vi "VXM-MoveOneAxisToHome.vi"(8 "error in (no error)":errorcluster, 9 "mmWave Axis to home":T1="RT3", 11 "Message que":T2) -> (0 "error out":errorcluster)   [LabVIEW 2019]
uses:
  Support/MessageQue/MessageQue.ctl
  Support/MessageQue/MessageCluster.ctl
  mmWaveAxis.ctl
  singleAxisMoveDef.ctl
  Support/MessageQue/MessageQue.lvlib
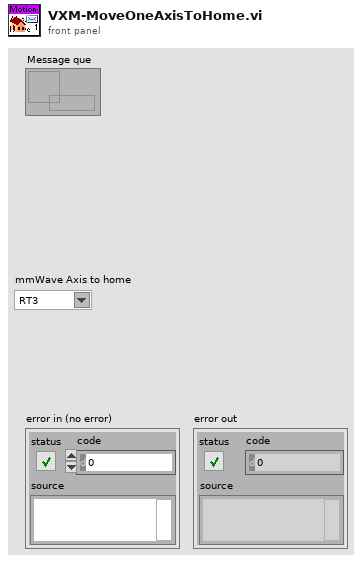
[diagram p1: front panel]
types:
  T1 = typedef "mmWaveAxis.ctl" = string
  T2 = typedef "MessageQue.lvlib/MessageQue.ctl" = refnum<queue>
  T3 = typedef "singleAxisMoveDef.ctl" = cluster{"mmWave Axis":T1, "eng. value":dbl}
  T4 = cluster{"Move Type":string, "Positions":T3[], "Position (Antenna or Raster)":i32, "Polarization":u16}
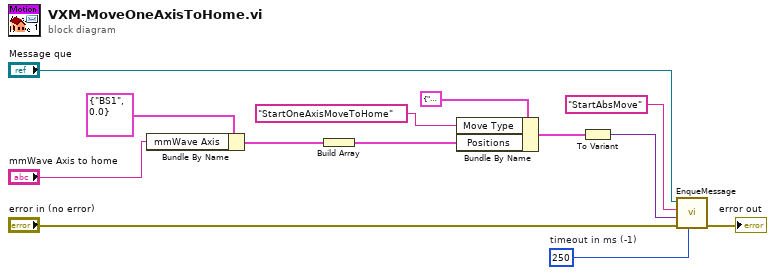
[diagram p0: block diagram]
diagram:
  w12 = 250  # timeout in ms (-1)
  n1 = Bundle By Name(cluster=T3 {"mmWave Axis"="BS1", "eng. value"=0.0} ("Move"), "mmWave Axis"="mmWave Axis to home") -> (w2:T3)
  n2 = Build Array(w2) -> (w1:T3[])
  n3 = Bundle By Name(cluster=T4 {"Move Type"="AllHomeMove", "Positions"=[], "Position (Antenna or Raster)"=0, "Polarization"=0} ("Move-Abs"), "Move Type"="StartOneAxisMoveToHome", "Positions"=w1) -> (w6:T4)
  n4 = To Variant(anything=w6) -> (Variant=w13:variant)
  n5 = call "EnqueMessage.vi"("timeout in ms (-1)"=w12, "error in"="error in (no error)", "Message Payload"=w13, "Message Command"="StartAbsMove", "Message que"="Message que") -> ("error out"=→"error out":errorcluster)  [unwired: 5 in, 1 out]
